vi "run.vi"(8 "error in (no error)":errorcluster, 11 "dotnet_system_exec in":refnum<class "dotnet_system_exec.lvclass">) -> (0 "error out":errorcluster, 3 "dotnet_system_exec out":refnum<class "dotnet_system_exec.lvclass">)   [LabVIEW 2013, in "dotnet_system_exec.lvclass"]
doc: "Runs the .NET System Process as configured with the @create method"
uses:
  dotnet_system_exec.lvclass
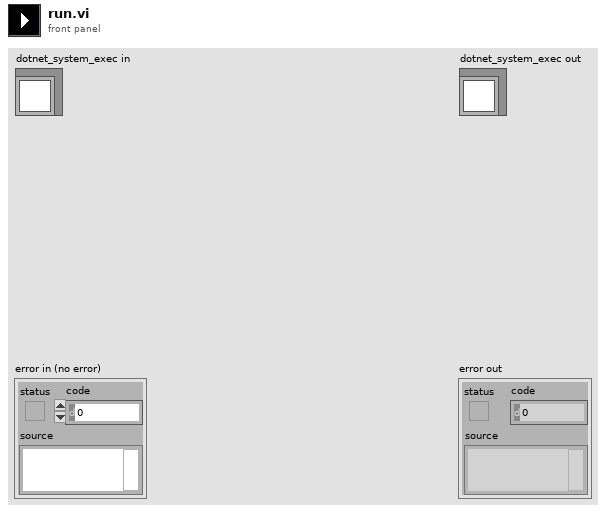
[diagram p1: front panel]
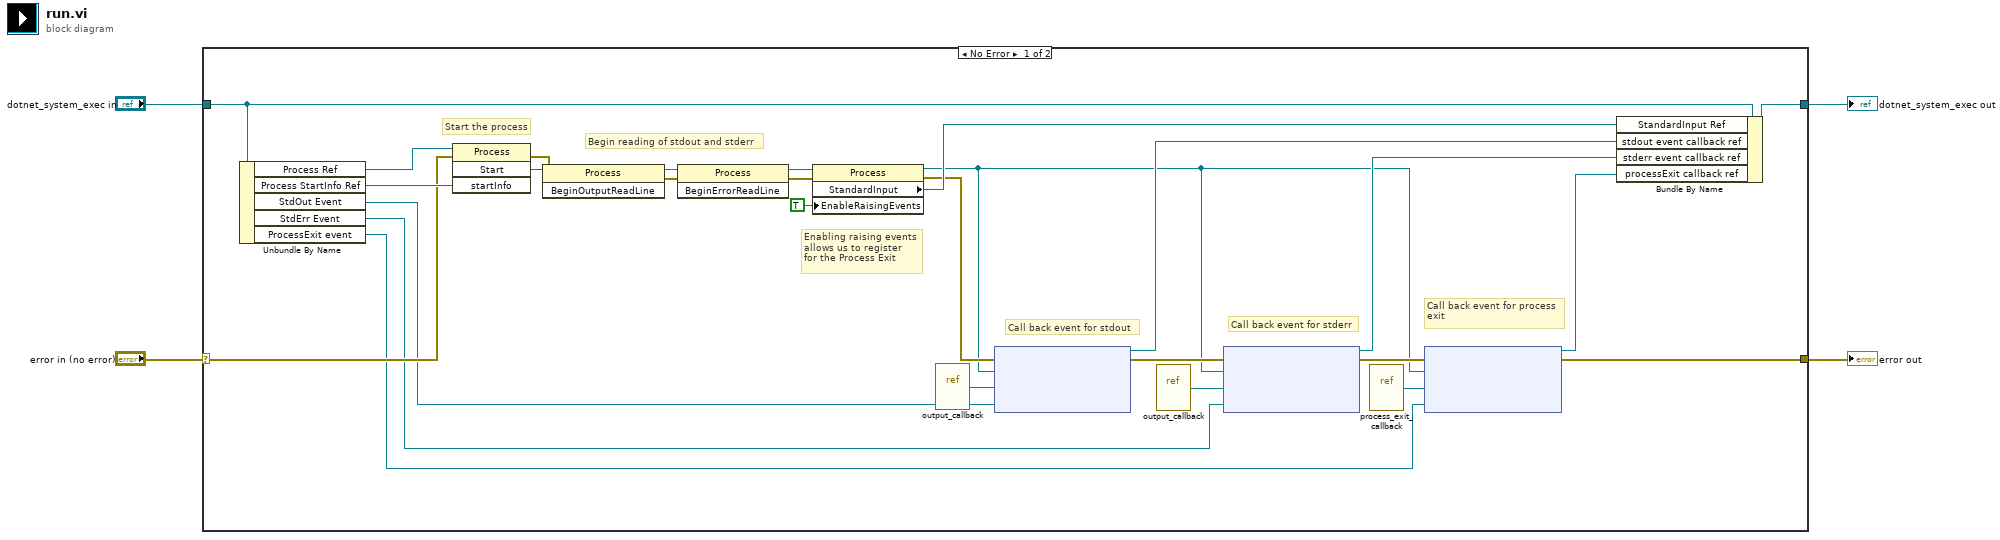
[diagram p0: block diagram]
diagram:
  n1 = case shown="No Error" "error in (no error)" {
    selector: "error in (no error)" -> [w23 w33]
    tunnel: [w8 w33] -> w3
    tunnel: [w16 w32] -> w1
    tunnel: "dotnet_system_exec in" -> [w22 w32]
    frame No Error {
      # "Call back event for process\nexit"
      # "Enabling raising events\nallows us to register\nfor the Process Exit"
      # "Call back event for stderr"
      # "Call back event for stdout"
      # "Begin reading of stdout and stderr"
      # "Start the process"
      n2 = Unbundle By Name(w22) -> ("Process Ref"=w29:refnum<k24>, "Process StartInfo Ref"=w28:refnum<k24>, "StdOut Event"=w20:refnum<user-event>, "StdErr Event"=w19:refnum<user-event>, "ProcessExit event"=w7:refnum<user-event>)
      n3 = invoke class="Process" method="Start"(reference=w29, error in=w23, "startInfo"=w28) -> (error out=w27:errorcluster, "Start"=w26:refnum<k24>)  [unwired: 1 in, 2 out]
      n4 = invoke class="Process" method="BeginOutputReadLine"(reference=w26, error in=w27) -> (reference out=w31:refnum<k24>, error out=w30:errorcluster)  [unwired: 1 in, 1 out]
      n5 = invoke class="Process" method="BeginErrorReadLine"(reference=w31, error in=w30) -> (reference out=w25:refnum<k24>, error out=w24:errorcluster)  [unwired: 1 in, 1 out]
      n6 = property class="Process"(reference=w25, error in=w24, "EnableRaisingEvents"=TRUE) -> (reference out=w9:refnum<k24>, error out=w18:errorcluster, "StandardInput"=w21:refnum<k24>)
      n7 = vi-ref "output_callback.vi"() -> ("vi reference"=w15:refnum<vi>)
      n8 = node(w18, w9, w15, w20) -> (w12:refnum<k27>, w17:errorcluster)  [unwired: 1 in]
      n9 = vi-ref "output_callback.vi"() -> ("vi reference"=w14:refnum<vi>)
      n10 = node(w17, w9, w14, w19) -> (w11:refnum<k27>, w10:errorcluster)  [unwired: 1 in]
      n11 = vi-ref "process_exit_callback.vi"() -> ("vi reference"=w6:refnum<vi>)
      n12 = node(w10, w9, w6, w7) -> (w5:refnum<k27>, w8:errorcluster)  [unwired: 1 in]
      n13 = Bundle By Name(cluster=w22, "StandardInput Ref"=w21, "stdout event callback ref"=w12, "stderr event callback ref"=w11, "processExit callback ref"=w5) -> (w16:refnum<class "dotnet_system_exec.lvclass">)
    }
    frame Error {
    }
  }
  "error out" <- w3
  "dotnet_system_exec out" <- w1
